vi "Close Sim.vi"(8 "error in (no error)":errorcluster, 11 "FPGA Sim in":refnum<class "FPGA Sim.lvclass">) -> (0 "error out":errorcluster)   [LabVIEW 2020, in "Unit Tests.lvlib" / "FPGA Sim.lvclass"]
uses:
  FPGA Sim.lvclass
  FPGA Sim.lvclass/FPGA Sim.ctl
  Dependencies/Virtual Memory Unit/Virtual Memory Unit.lvclass
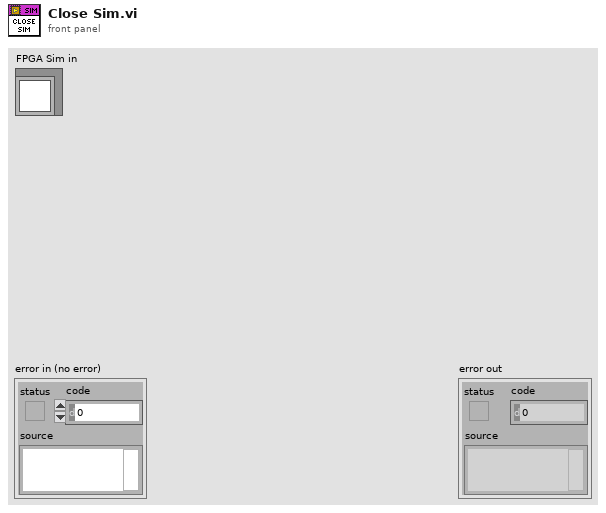
[diagram p1: front panel]
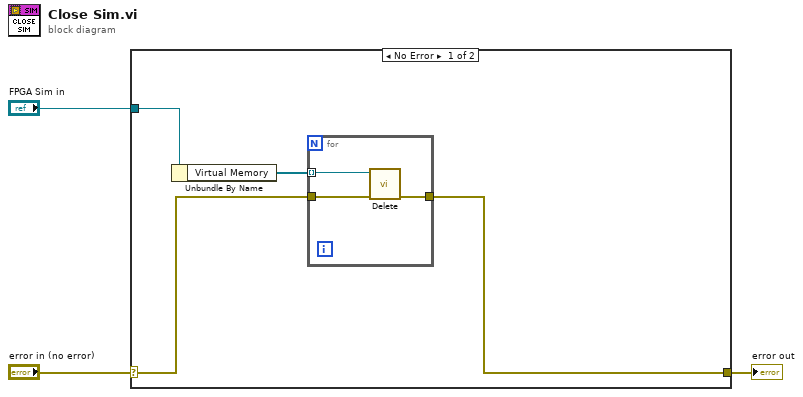
[diagram p0: block diagram]
diagram:
  n1 = case shown="No Error" "error in (no error)" {
    selector: "error in (no error)" -> [w5 w11]
    tunnel: [w4 w11] -> w2
    tunnel: "FPGA Sim in" -> [w7 _]
    frame No Error {
      n2 = Unbundle By Name(w7) -> ("Virtual Memory"=w6:refnum<class "Virtual Memory Unit.lvclass">[])
      n3 = for {
        tunnel: w6 -> [w10] mode=indexing
        tunnel: w5 -> [w9]
        tunnel: [w8] -> w4
        n4 = call "Delete.vi"("error in (no error)"=w9, "Virtual Memory Unit in"=w10) -> ("error out"=w8:errorcluster)  [unwired: 9 in]
      }
    }
    frame Error {
    }
  }
  "error out" <- w2
